vi "Test 6.vi"() -> ()   [LabVIEW 2019]
panel:
  in  "数值 3":fxp<+,2,2>
  out "溢出？":bool
  out "数值 2":fxp<+,2,2>
  in  "数值":fxp<+,2,2>
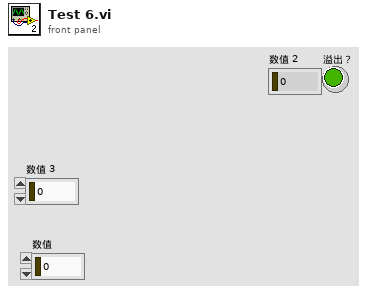
[diagram p1: front panel]
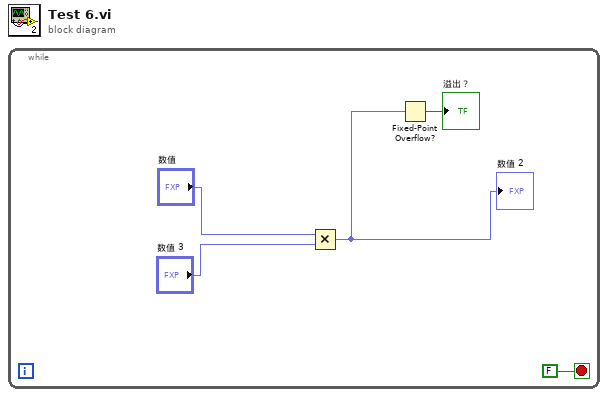
[diagram p0: block diagram]
diagram:
  n1 = while {
    stop <- FALSE stop-if-true
    n2 = Multiply(x="数值", y="数值 3") -> (x*y=w2:fxp<+,4,4>)
    "数值 2" <- w2
    n3 = Fixed-Point Overflow?(1:w2) -> (0:→"溢出？":bool)
  }
